vi "FFTBoost.vi"(7 "CompensationCoefficients":dbl[](array[numeric])=[1.0, 1.0, 0.0, 0.0, 0.0], 10 "mutedData":dbl[](array[numeric])=array[1605632 elements], 11 "SamplingFreq (for graph)":dbl=500.0) -> (2 "boostedData":dbl[](array[numeric]))   [LabVIEW 2011]
uses:
  <vilib>/Analysis/2dsp.llb/Real FFT.vi
  <vilib>/Analysis/2dsp.llb/Inverse Real FFT.vi
  <vilib>/Analysis/NI_AALPro.lvlib
panel:
  out "Waveform Graph":cluster{i32, dbl, dbl[]}[](graph)
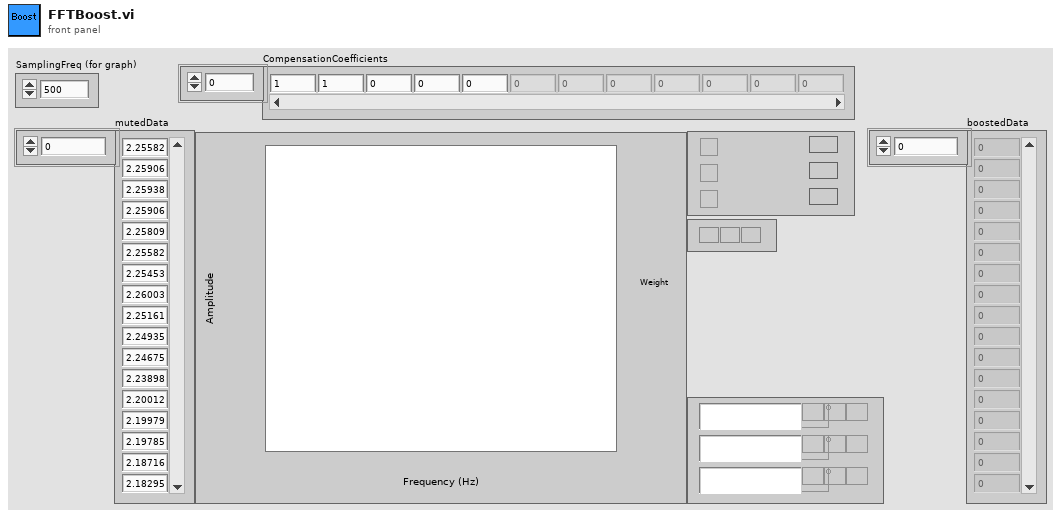
[diagram p1: front panel]
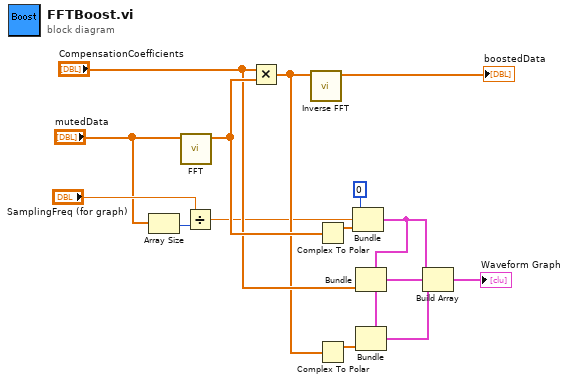
[diagram p0: block diagram]
diagram:
  n1 = Array Size(array="mutedData") -> (size(s)=w4:i32)
  n2 = call-poly <vilib>:"FFT.vi"("X"="mutedData") -> ("FFT {X}"=w14:cdb[])  [unwired: 2 in, 8 out]
  n3 = Divide(x="SamplingFreq (for graph)", y=w4) -> (x/y=w3:dbl)
  n4 = Multiply(x="CompensationCoefficients", y=w14) -> (x*y=w7:cdb[])
  n5 = call-poly <vilib>:"Inverse FFT.vi"("FFT {X}"=w7) -> ("X"=→"boostedData":dbl[])  [unwired: 1 in, 9 out]
  n6 = Complex To Polar(r * e^(i*theta)=w14) -> (r=w13:dbl[])  [unwired: 1 out]
  n7 = Complex To Polar(r * e^(i*theta)=w7) -> (r=w6:dbl[])  [unwired: 1 out]
  n8 = Bundle(0, w3, w13) -> (w10:cluster{i32, dbl, dbl[]})  [unwired: 1 in]
  n9 = Bundle(cluster=w10, "CompensationCoefficients") -> (w12:cluster{i32, dbl, dbl[]})  [unwired: 2 in]
  n10 = Bundle(cluster=w10, w6) -> (w11:cluster{i32, dbl, dbl[]})  [unwired: 2 in]
  n11 = Build Array(w10, w12, w11) -> (→"Waveform Graph":cluster{i32, dbl, dbl[]}[])
